vi "DC Gap (1 Ch).vi"(8 "error in (no error)":errorcluster, 11 "Waveform":waveform(sgl)) -> (0 "error out":errorcluster, 1 "DC gap":sgl, 2 "AC coupled wfm":waveform(sgl))   [LabVIEW 2017, in "VibrationAnalysisFunctions.lvlib"]
doc: "Calculates DC gap in EU.\nAC couples the original waveform."
uses:
  <vilib>/addons/InsightCM/Utilities/Analysis/Vibration/VibrationAnalysisFunctions.lvlib
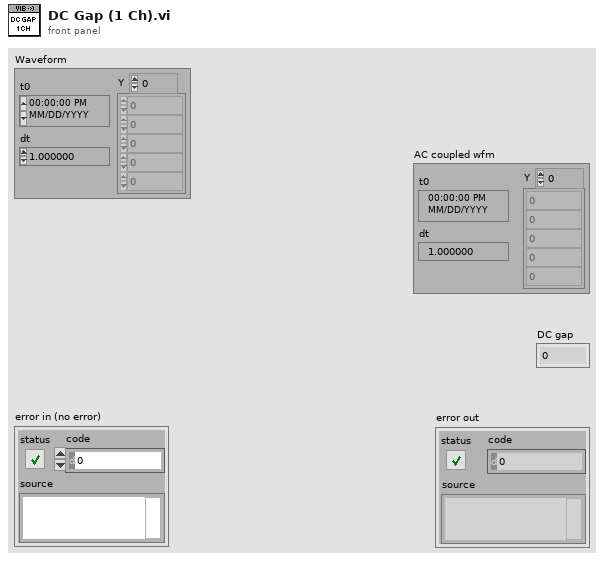
[diagram p1: front panel]
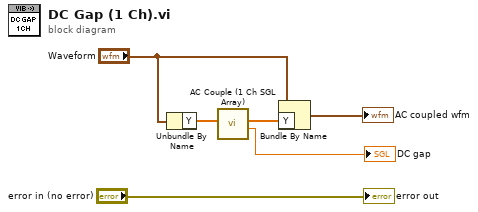
[diagram p0: block diagram]
diagram:
  n1 = Unbundle By Name("Waveform") -> ("Y"=w2:sgl[])
  n2 = call <vilib>:"AC Couple (1 Ch SGL Array).vi"("Signal"=w2) -> ("DC"=→"DC gap":sgl, "AC Coupled"=w5:sgl[])  [unwired: 8 in, 1 out]
  n3 = Bundle By Name(cluster="Waveform", "Y"=w5) -> (→"AC coupled wfm":waveform(sgl))
  "error out" <- "error in (no error)"
